vi "Kinesis-Microestruturacao-Circuits.vi"() -> ()   [LabVIEW 2014]
doc: "André Romero - 2017\nandretec@ifsc.usp.br"
uses:
  C:/UserLab/andre/GITs/andretec/Thorlabs-Vector-Move/kinesisTec/Kinesis/Thorlabs.MotionControl.Controls.dll
  Kinesis/Thorlabs.MotionControl.Controls.dll
  Basic-VIs/motorsGlobalVar.vi
  <vilib>/Instr/_visa.llb/VISA Configure Serial Port (Instr).vi
panel:
  in  "Raio":dbl=0.01
  in  "Density":dbl=100.0
  in  "Adjust Motors":bool
  out "Process time":string="0:00:50"
  out "Progress %":dbl(slide) scale=0.0..100.0
  out "XY Graph":cluster{"Graph X":dbl[], "Graph Y":dbl[]}(graph)
  in  "Swap XY":bool
  out "stop cronometro":bool=TRUE
  in  "Stop Button":bool
  in  "Graph Y":dbl[](array[numeric])=[0.0, 0.0, 6.6674440298507465, 6.6674440298507465, 6.6674440298507465, 6.6674440298507465, 6.6674440298507465, 6.6674440298507465, 6.6674440298507465, 6.6674440298507465, 6.6674440298507465, 6.6674440298507465, 6.6674440298507465, 6.6674440298507465, 6.6674440298507465, 6.6674440298507465, 6.6674440298507465, 6.6674440298507465, 6.6674440298507465, 6.6674440298507465, 6.6674440298507465, 6.6674440298507465, 6.6674440298507465, 6.6674440298507465, 6.6674440298507465, 6.6674440298507465, 6.6674440298507465, 6.6674440298507465, 6.6674440298507465, 6.6674440298507465, 6.6674440298507465, 6.6674440298507465, 6.6674440298507465, 6.6674440298507465, 6.6674440298507465, 6.6674440298507465, 6.6674440298507465, 6.6674440298507465, 6.6674440298507465, 6.6674440298507465, 6.6674440298507465, 6.6674440298507465, 6.6674440298507465, 6.673128498134329, 6.673128498134329, 6.673128498134329, 6.673128498134329, 6.673128498134329, 6.687354244402985, 6.687354244402985, 6.687354244402985, 6.687354244402985, 6.687354244402985, 6.692543143656716, 6.692543143656716, 6.692543143656716, 6.692543143656716, 6.692543143656716, 6.692543143656716, 6.692543143656716, 6.692543143656716, 6.692543143656716, 6.692543143656716, 6.692543143656716, 6.692543143656716, 6.691522854477612, 6.691522854477612, 6.691522854477612, 6.691522854477612, 6.691522854477612, 6.680183069029851, 6.680183069029851, 6.680183069029851, 6.680183069029851, 6.680183069029851, 6.658640391791045, 6.658640391791045, 6.658640391791045, 6.658640391791045, 6.658640391791045, 6.644793610074627, 6.644793610074627, 6.644793610074627, 6.644793610074627, 6.644793610074627, 6.642490671641791, 6.642490671641791, 6.642490671641791, 6.642490671641791, 6.642490671641791, 6.642490671641791, 6.642490671641791, 6.642490671641791, 6.642490671641791, 6.642490671641791, 6.642490671641791, 6.642490671641791, 6.642490671641791, 6.642490671641791, 6.642490671641791, 6.647825326492537, 6.647825326492537, 6.647825326492537, 6.647825326492537, 6.647825326492537, 6.66543260261194, 6.66543260261194, 6.66543260261194, 6.66543260261194, 6.66543260261194, 6.685226212686567, 6.685226212686567, 6.685226212686567, 6.685226212686567, 6.685226212686567, 6.692484841417911, 6.692484841417911, 6.692484841417911, 6.692484841417911, 6.692484841417911, 6.692543143656716, 6.692543143656716, 6.692543143656716, 6.692543143656716, 6.692543143656716, 6.692543143656716, 6.692543143656716, 6.691464552238806, 6.691464552238806, 6.691464552238806, 6.691464552238806, 6.691464552238806, 6.679833255597015, 6.679833255597015, 6.679833255597015, 6.679833255597015, 6.679833255597015, 6.658057369402985, 6.658057369402985, 6.658057369402985, 6.658057369402985, 6.658057369402985, 6.644647854477612, 6.644647854477612, 6.644647854477612, 6.644647854477612, 6.644647854477612, 6.642548973880597, 6.642548973880597, 6.642548973880597, 6.642548973880597, 6.642548973880597, 6.642519822761194, 6.642519822761194, 6.642519822761194, 6.642519822761194, 6.642519822761194, 6.642519822761194, 6.642519822761194, 6.642519822761194, 6.643569263059701, 6.643569263059701, 6.643569263059701, 6.643569263059701, 6.643569263059701, 6.655521222014926, 6.655521222014926, 6.655521222014926, 6.655521222014926, 6.655521222014926, 6.677180503731344, 6.677180503731344, 6.677180503731344, 6.677180503731344, 6.677180503731344, 6.690531716417911, 6.690531716417911, 6.690531716417911, 6.690531716417911, 6.690531716417911, 6.692572294776119, 6.692572294776119, 6.692572294776119, 6.692572294776119, 6.692572294776119, 6.692572294776119, 6.692572294776119, 6.692572294776119, 6.692572294776119, 6.692572294776119, 6.692572294776119, 6.692572294776119, 6.691522854477612, 6.691522854477612, 6.691522854477612, 6.691522854477612, 6.691522854477612, 6.680008162313433, 6.680008162313433, 6.680008162313433, 6.680008162313433, 6.680008162313433, 6.668668376865671, 6.668668376865671, 6.668668376865671, 6.668668376865671, 6.668668376865671, 6.667502332089552, 6.667502332089552, 6.667502332089552, 6.667502332089552, 6.667502332089552, 6.667502332089552, 6.667502332089552, 6.667502332089552, 6.667502332089552, 6.667502332089552, 6.667502332089552, 6.667502332089552, 6.667531483208955, 6.667531483208955, 6.667531483208955, 6.667531483208955, 6.667531483208955, 6.667531483208955, 6.667531483208955, 6.667531483208955, 6.667531483208955, 6.667531483208955, 6.667531483208955, 6.667531483208955, 6.667531483208955, 6.667531483208955, 6.667531483208955, 6.667531483208955, 6.667531483208955, 6.667531483208955, 6.667531483208955, 6.667531483208955, 6.667531483208955, 6.667531483208955, 6.667531483208955, 6.667531483208955, 6.667531483208955, 6.667531483208955, 6.667531483208955, 6.667531483208955, 6.667531483208955, 6.667531483208955, 6.667531483208955, 6.667531483208955, 6.667531483208955, 6.667531483208955, 6.667531483208955, 6.667531483208955, 6.667531483208955, 6.6663945895522385, 6.6663945895522385, 6.6663945895522385, 6.6663945895522385, 6.6663945895522385, 6.662051072761194, 6.662051072761194, 6.662051072761194, 6.662051072761194, 6.662051072761194, 6.644035680970149, 6.644035680970149, 6.644035680970149, 6.644035680970149, 6.644035680970149, 6.606430736940299, 6.606430736940299, 6.606430736940299, 6.606430736940299, 6.606430736940299, 6.593924906716418, 6.593924906716418, 6.593924906716418, 6.593924906716418, 6.593924906716418, 6.574539412313433, 6.574539412313433, 6.574539412313433, 6.574539412313433, 6.574539412313433, 6.567484841417911, 6.567484841417911, 6.567484841417911, 6.567484841417911, 6.567484841417911, 6.567484841417911, 6.567484841417911, 6.567484841417911, 6.567484841417911, 6.567484841417911, 6.567484841417911, 6.567513992537314, 6.567513992537314, 6.567513992537314, 6.567513992537314, 6.567513992537314, 6.567513992537314, 6.567513992537314, 6.567513992537314, 6.567513992537314, 6.567513992537314, 6.567543143656716, 6.567543143656716, 6.567543143656716, 6.567543143656716, 6.567543143656716, 6.567543143656716, 6.567543143656716, 6.567543143656716, 6.567543143656716, 6.567543143656716, 6.567543143656716, 6.567543143656716, 6.567543143656716, 6.567543143656716, 6.567543143656716, 6.567543143656716, 6.567543143656716, 6.567543143656716, 6.567543143656716, 6.567543143656716, 6.567543143656716, 6.567543143656716, 6.567543143656716, 6.567543143656716, 6.567543143656716, 6.567543143656716, 6.567543143656716, 6.567543143656716, 6.567543143656716, 6.567543143656716, 6.567543143656716, 6.567543143656716, 6.567543143656716, 6.567543143656716, 6.567543143656716, 6.567543143656716, 6.567543143656716, 6.567543143656716, 6.567543143656716, 6.567543143656716, 6.567543143656716, 6.567543143656716, 6.567543143656716, 6.567543143656716, 6.567543143656716, 6.567543143656716, 6.567543143656716, 6.567543143656716, 6.567543143656716, 6.567543143656716, 6.567543143656716, 6.567543143656716, 6.567543143656716, 6.567543143656716, 6.5667852145522385, 6.5667852145522385, 6.5667852145522385, 6.5667852145522385, 6.5667852145522385, 6.555299673507463, 6.555299673507463, 6.555299673507463, 6.555299673507463, 6.555299673507463, 6.533523787313433, 6.533523787313433, 6.533523787313433, 6.533523787313433, 6.533523787313433, 6.525186567164179, 6.525186567164179, 6.525186567164179, 6.525186567164179, 6.525186567164179, 6.517490671641791, 6.517490671641791, 6.517490671641791, 6.517490671641791, 6.517490671641791, 6.517490671641791, 6.517490671641791, 6.517490671641791, 6.517490671641791, 6.517490671641791, 6.517519822761194, 6.517519822761194, 6.517519822761194, 6.517519822761194, 6.517519822761194, 6.517519822761194, 6.517519822761194, 6.517519822761194, 6.517519822761194, 6.517519822761194, 6.517548973880597, 6.517548973880597, 6.517548973880597, 6.517548973880597, 6.517548973880597, 6.517548973880597, 6.517548973880597, 6.517548973880597, 6.517548973880597, 6.517548973880597, 6.517548973880597, 6.517548973880597, 6.517548973880597, 6.517548973880597, 6.517548973880597, 6.517548973880597, 6.517548973880597, 6.517548973880597, 6.517548973880597, 6.517548973880597, 6.517548973880597, 6.517548973880597, 6.517548973880597, 6.517548973880597, 6.517548973880597, 6.517548973880597, 6.517548973880597, 6.517548973880597, 6.517548973880597, 6.517548973880597, 6.517548973880597, 6.517548973880597, 6.517548973880597, 6.517548973880597, 6.517548973880597, 6.517548973880597, 6.517548973880597, 6.517548973880597, 6.517548973880597, 6.517548973880597, 6.517548973880597, 6.517548973880597, 6.517548973880597, 6.517548973880597, 6.517548973880597, 6.517548973880597, 6.517548973880597, 6.517548973880597, 6.517548973880597, 6.517548973880597, 6.517548973880597, 6.517548973880597, 6.517548973880597, 6.517548973880597, 6.517548973880597, 6.517548973880597, 6.517548973880597, 6.517548973880597, 6.517548973880597, 6.517548973880597, 6.516674440298507, 6.516674440298507, 6.516674440298507, 6.516674440298507, 6.516674440298507, 6.504897388059701, 6.504897388059701, 6.504897388059701, 6.504897388059701, 6.504897388059701, 6.481926305970149, 6.481926305970149, 6.481926305970149, 6.481926305970149, 6.481926305970149, 6.456943796641791, 6.456943796641791, 6.456943796641791, 6.456943796641791, 6.456943796641791, 6.4330690298507465, 6.4330690298507465, 6.4330690298507465, 6.4330690298507465, 6.4330690298507465, 6.419717817164179, 6.419717817164179, 6.419717817164179, 6.419717817164179, 6.419717817164179, 6.417473180970149, 6.417473180970149, 6.417473180970149, 6.417473180970149, 6.417473180970149, 6.417473180970149]
  in  "Graph X":dbl[](array[numeric])=[0.0, 0.0, 3.605935167910448, 3.605935167910448, 3.605935167910448, 3.605935167910448, 3.605935167910448, 3.609987173507463, 3.609987173507463, 3.609987173507463, 3.609987173507463, 3.609987173507463, 3.627157182835821, 3.627157182835821, 3.627157182835821, 3.627157182835821, 3.627157182835821, 3.6520813899253732, 3.6520813899253732, 3.6520813899253732, 3.6520813899253732, 3.6520813899253732, 3.6770930503731343, 3.6770930503731343, 3.6770930503731343, 3.6770930503731343, 3.6770930503731343, 3.697323927238806, 3.697323927238806, 3.697323927238806, 3.697323927238806, 3.697323927238806, 3.705311333955224, 3.705311333955224, 3.705311333955224, 3.705311333955224, 3.705311333955224, 3.705311333955224, 3.705311333955224, 3.705311333955224, 3.705311333955224, 3.705311333955224, 3.705311333955224, 3.7063024720149254, 3.7063024720149254, 3.7063024720149254, 3.7063024720149254, 3.7063024720149254, 3.7175839552238807, 3.7175839552238807, 3.7175839552238807, 3.7175839552238807, 3.7175839552238807, 3.7291861007462686, 3.7291861007462686, 3.7291861007462686, 3.7291861007462686, 3.7291861007462686, 3.7303521455223883, 3.7303521455223883, 3.7303521455223883, 3.7303521455223883, 3.7303521455223883, 3.7303521455223883, 3.7303521455223883, 3.7303521455223883, 3.7303521455223883, 3.7303521455223883, 3.7303521455223883, 3.7303521455223883, 3.7366779384328357, 3.7366779384328357, 3.7366779384328357, 3.7366779384328357, 3.7366779384328357, 3.7554221082089554, 3.7554221082089554, 3.7554221082089554, 3.7554221082089554, 3.7554221082089554, 3.774137126865672, 3.774137126865672, 3.774137126865672, 3.774137126865672, 3.774137126865672, 3.7803463152985075, 3.7803463152985075, 3.7803463152985075, 3.7803463152985075, 3.7803463152985075, 3.7803463152985075, 3.7803463152985075, 3.7803463152985075, 3.7803463152985075, 3.7803463152985075, 3.7803463152985075, 3.7803463152985075, 3.7803463152985075, 3.7803463152985075, 3.7803463152985075, 3.781803871268657, 3.781803871268657, 3.781803871268657, 3.781803871268657, 3.781803871268657, 3.7941930970149254, 3.7941930970149254, 3.7941930970149254, 3.7941930970149254, 3.7941930970149254, 3.816027285447761, 3.816027285447761, 3.816027285447761, 3.816027285447761, 3.816027285447761, 3.828678871268657, 3.828678871268657, 3.828678871268657, 3.828678871268657, 3.828678871268657, 3.8303404850746268, 3.8303404850746268, 3.8303404850746268, 3.8303404850746268, 3.8303404850746268, 3.8303404850746268, 3.8303404850746268, 3.8303404850746268, 3.8303404850746268, 3.8303404850746268, 3.8303404850746268, 3.8303404850746268, 3.8368703358208953, 3.8368703358208953, 3.8368703358208953, 3.8368703358208953, 3.8368703358208953, 3.8447994402985075, 3.8447994402985075, 3.8447994402985075, 3.8447994402985075, 3.8447994402985075, 3.866633628731343, 3.866633628731343, 3.866633628731343, 3.866633628731343, 3.866633628731343, 3.8803346548507465, 3.8803346548507465, 3.8803346548507465, 3.8803346548507465, 3.8803346548507465, 3.8803346548507465, 3.8803346548507465, 3.8803346548507465, 3.8803346548507465, 3.8803346548507465, 3.8803346548507465, 3.8803346548507465, 3.8803346548507465, 3.8803346548507465, 3.8803346548507465, 3.8803346548507465, 3.8803346548507465, 3.8803346548507465, 3.886631296641791, 3.886631296641791, 3.886631296641791, 3.886631296641791, 3.886631296641791, 3.9054046175373136, 3.9054046175373136, 3.9054046175373136, 3.9054046175373136, 3.9054046175373136, 3.92411963619403, 3.92411963619403, 3.92411963619403, 3.92411963619403, 3.92411963619403, 3.9303288246268657, 3.9303288246268657, 3.9303288246268657, 3.9303288246268657, 3.9303288246268657, 3.9303288246268657, 3.9303288246268657, 3.9303288246268657, 3.9303288246268657, 3.9303288246268657, 3.9303288246268657, 3.9303288246268657, 3.9303288246268657, 3.9303288246268657, 3.9303288246268657, 3.9303288246268657, 3.9303288246268657, 3.936800373134328, 3.936800373134328, 3.936800373134328, 3.936800373134328, 3.936800373134328, 3.9445545708955225, 3.9445545708955225, 3.9445545708955225, 3.9445545708955225, 3.9445545708955225, 3.95536963619403, 3.95536963619403, 3.95536963619403, 3.95536963619403, 3.95536963619403, 3.95536963619403, 3.95536963619403, 3.95536963619403, 3.95536963619403, 3.95536963619403, 3.95536963619403, 3.95536963619403, 3.956652285447761, 3.956652285447761, 3.956652285447761, 3.956652285447761, 3.956652285447761, 3.961141557835821, 3.961141557835821, 3.961141557835821, 3.961141557835821, 3.961141557835821, 3.9795067630597014, 3.9795067630597014, 3.9795067630597014, 3.9795067630597014, 3.9795067630597014, 4.004518423507463, 4.004518423507463, 4.004518423507463, 4.004518423507463, 4.004518423507463, 4.0406366604477615, 4.0406366604477615, 4.0406366604477615, 4.0406366604477615, 4.0406366604477615, 4.048624067164179, 4.048624067164179, 4.048624067164179, 4.048624067164179, 4.048624067164179, 4.0553579757462686, 4.0553579757462686, 4.0553579757462686, 4.0553579757462686, 4.0553579757462686, 4.0553579757462686, 4.0553579757462686, 4.055387126865671, 4.055387126865671, 4.055387126865671, 4.055387126865671, 4.055387126865671, 4.055387126865671, 4.055387126865671, 4.055387126865671, 4.055387126865671, 4.055387126865671, 4.0553579757462686, 4.0553579757462686, 4.0553579757462686, 4.0553579757462686, 4.0553579757462686, 4.0553579757462686, 4.0553579757462686, 4.0553579757462686, 4.0553579757462686, 4.0553579757462686, 4.0553579757462686, 4.0553579757462686, 4.0553579757462686, 4.0553579757462686, 4.0553579757462686, 4.0553579757462686, 4.0553579757462686, 4.0553579757462686, 4.0553579757462686, 4.0553579757462686, 4.0553579757462686, 4.0553579757462686, 4.0553579757462686, 4.0553579757462686, 4.0553579757462686, 4.0553579757462686, 4.0553579757462686, 4.0553579757462686, 4.0553579757462686, 4.0553579757462686, 4.0553579757462686, 4.061800373134329, 4.061800373134329, 4.061800373134329, 4.061800373134329, 4.061800373134329, 4.06972947761194, 4.06972947761194, 4.06972947761194, 4.06972947761194, 4.06972947761194, 4.091534514925373, 4.091534514925373, 4.091534514925373, 4.091534514925373, 4.091534514925373, 4.105352145522388, 4.105352145522388, 4.105352145522388, 4.105352145522388, 4.105352145522388, 4.105381296641791, 4.105381296641791, 4.105381296641791, 4.105381296641791, 4.105381296641791, 4.105381296641791, 4.105381296641791, 4.1050897854477615, 4.1050897854477615, 4.1050897854477615, 4.1050897854477615, 4.1050897854477615, 4.0951784048507465, 4.0951784048507465, 4.0951784048507465, 4.0951784048507465, 4.0951784048507465, 4.073489972014926, 4.073489972014926, 4.073489972014926, 4.073489972014926, 4.073489972014926, 4.060954990671642, 4.060954990671642, 4.060954990671642, 4.060954990671642, 4.060954990671642, 4.023874766791045, 4.023874766791045, 4.023874766791045, 4.023874766791045, 4.023874766791045, 4.008687033582089, 4.008687033582089, 4.008687033582089, 4.008687033582089, 4.008687033582089, 4.005363805970149, 4.005363805970149, 4.005363805970149, 4.005363805970149, 4.005363805970149, 4.005363805970149, 4.005363805970149, 4.005363805970149, 4.005363805970149, 4.005363805970149, 4.005363805970149, 4.005363805970149, 4.005363805970149, 4.005363805970149, 4.005363805970149, 4.005363805970149, 4.005363805970149, 4.005392957089552, 4.005392957089552, 4.005392957089552, 4.005392957089552, 4.005392957089552, 4.005392957089552, 4.005392957089552, 4.005392957089552, 4.005392957089552, 4.005392957089552, 4.005392957089552, 4.005392957089552, 4.005392957089552, 4.005392957089552, 4.005392957089552, 4.005392957089552, 4.005392957089552, 4.005392957089552, 4.005392957089552, 4.005392957089552, 4.011631296641791, 4.011631296641791, 4.011631296641791, 4.011631296641791, 4.011631296641791, 4.019472947761194, 4.019472947761194, 4.019472947761194, 4.019472947761194, 4.019472947761194, 4.042852145522388, 4.042852145522388, 4.042852145522388, 4.042852145522388, 4.042852145522388, 4.080398787313433, 4.080398787313433, 4.080398787313433, 4.080398787313433, 4.080398787313433, 4.099113805970149, 4.099113805970149, 4.099113805970149, 4.099113805970149, 4.099113805970149, 4.103777985074627, 4.103777985074627, 4.103777985074627, 4.103777985074627, 4.103777985074627, 4.105410447761194, 4.105410447761194, 4.105410447761194, 4.105410447761194, 4.105410447761194, 4.105410447761194, 4.105410447761194, 4.105410447761194, 4.105381296641791, 4.105381296641791, 4.105381296641791, 4.105381296641791, 4.105381296641791, 4.098297574626866, 4.098297574626866, 4.098297574626866, 4.098297574626866, 4.098297574626866, 4.089989505597015, 4.089989505597015, 4.089989505597015, 4.089989505597015, 4.089989505597015, 4.06083838619403, 4.06083838619403, 4.06083838619403, 4.06083838619403, 4.06083838619403, 4.0553579757462686, 4.0553579757462686, 4.0553579757462686, 4.0553579757462686, 4.0553579757462686, 4.0553579757462686, 4.0553579757462686, 4.0553579757462686, 4.0553579757462686, 4.0553579757462686, 4.0553579757462686, 4.0553579757462686, 4.055387126865671, 4.055387126865671, 4.055387126865671, 4.055387126865671, 4.055387126865671, 4.055416277985074, 4.055416277985074, 4.055416277985074, 4.055416277985074, 4.055416277985074, 4.055416277985074, 4.055416277985074, 4.055416277985074, 4.055416277985074, 4.055416277985074, 4.055416277985074, 4.055416277985074, 4.055416277985074, 4.055416277985074, 4.055416277985074, 4.055416277985074, 4.055416277985074, 4.055416277985074, 4.055416277985074, 4.055416277985074, 4.055416277985074, 4.055416277985074, 4.055416277985074, 4.055416277985074, 4.055416277985074, 4.055416277985074, 4.055416277985074, 4.055416277985074, 4.055416277985074, 4.055416277985074, 4.055416277985074]
  out "GetPOS Y":dbl=6.417473180970149 format="%_6f"
  out "GetPOS X":dbl=4.055416277985074 format="%#_6f"
  out ".NET Refnum out 2":refnum<k24>
  out ".NET Refnum out 1":refnum<k24>
  out "Motor 2":bool
  out "Motor 1":bool
  in  "Acceleration (mm/s)":dbl=0.05
  in  "Iniciar":bool
  in  "Velocity (mm/s)":sgl=0.05
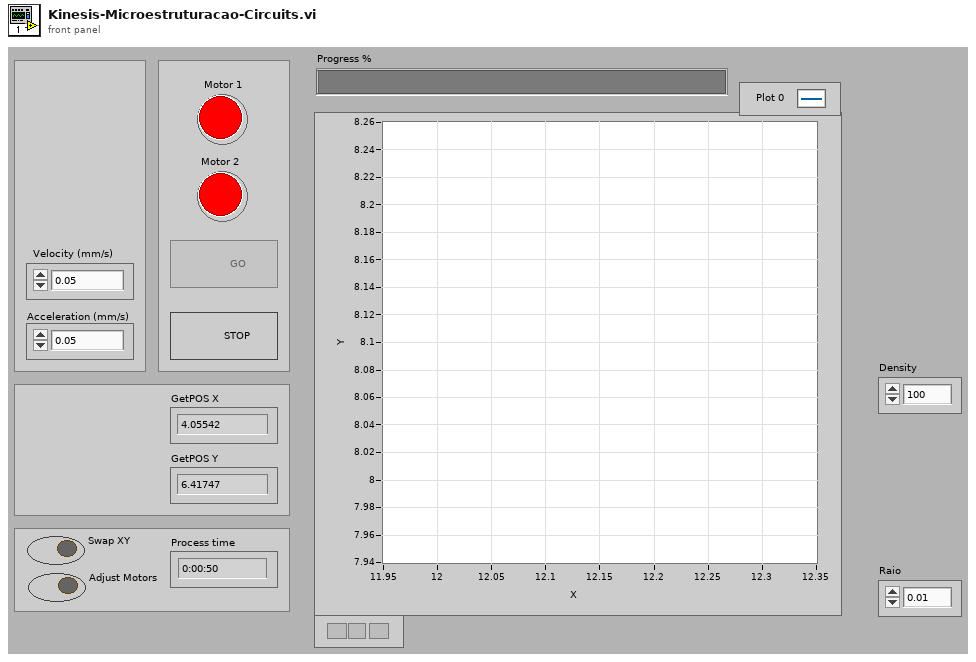
[diagram p1: front panel]
types:
  T1 = enum8{"Enabled", "Disabled", "Disabled and Grayed Out"}
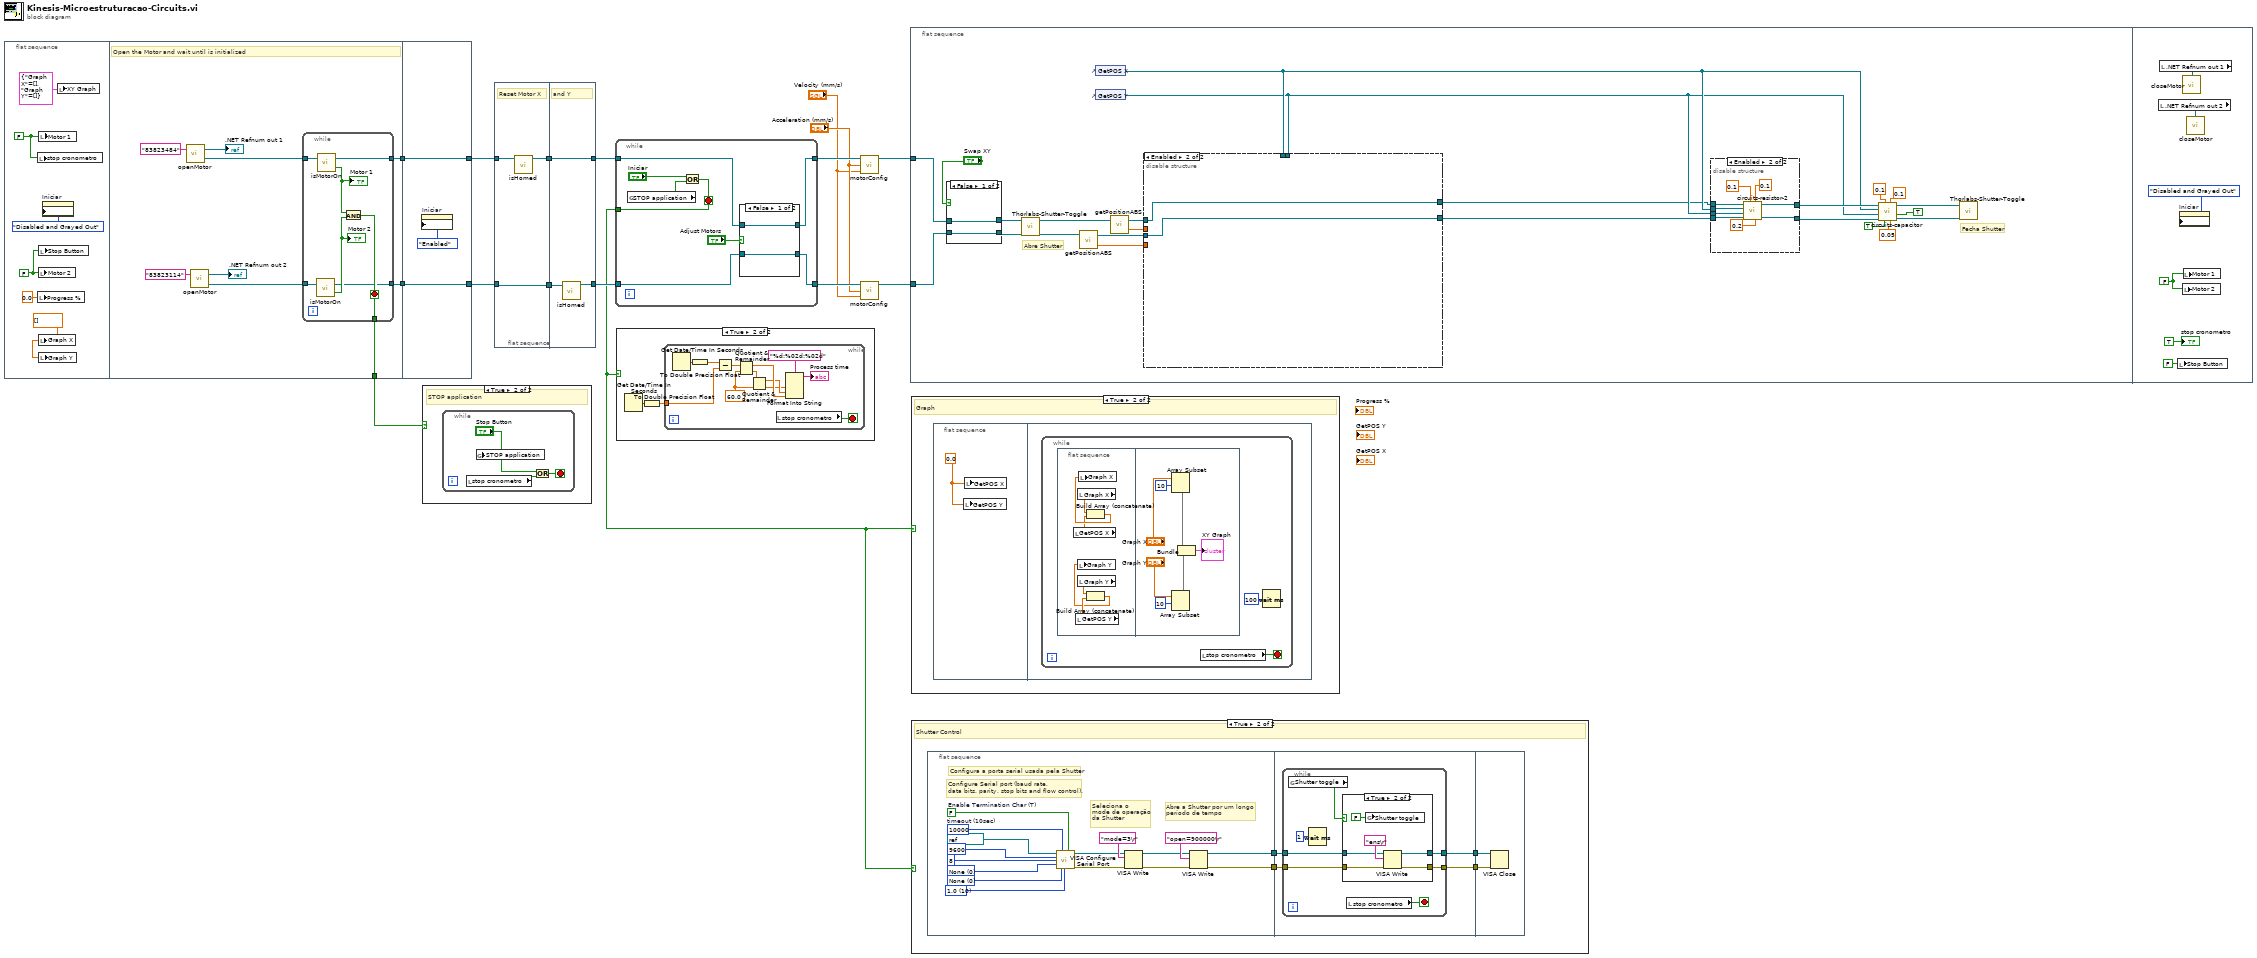
[diagram p0: block diagram]
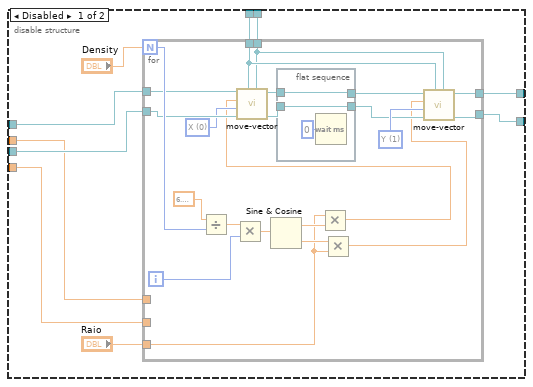
[diagram p6: hidden frame]
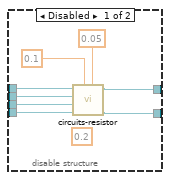
[diagram p7: hidden frame]
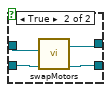
[diagram p8: hidden frame]
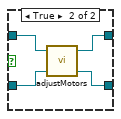
[diagram p10: hidden frame]
diagram:
  n1 = flat-sequence {
    tunnel: [w31] -> w4
    tunnel: [w30] -> w3
    tunnel: [w29] -> w2
    tunnel: [w40] -> w7
    tunnel: [w41] -> w8
    tunnel: w4 -> [w41]
    tunnel: w3 -> [w40]
    frame #0 {
      w18 = dbl[] [] ("Graph Y")
      w21 = FALSE ("Motor3\nLigado")
      w22 = FALSE
      n2 = local write "stop cronometro"(w22) -> ()
      n3 = local write "Progress %"(0.0 ("Progress %")) -> ()
      n4 = local write "Motor 2"(w21) -> ()
      n5 = local write "Graph X"(w18) -> ()
      n6 = local write "Motor 1"(w22) -> ()
      n7 = local write "Stop Button"(w21) -> ()
      n8 = local write "Graph Y"(w18) -> ()
      n9 = property on="Iniciar" class="Bool (strict)"("DisabledEnum"=T1."Disabled and Grayed Out" ("Disabled")) -> ()  [unwired: 2 in, 2 out]
      n10 = local write "XY Graph"(cluster{"Graph X":dbl[], "Graph Y":dbl[]} {"Graph X"=[], "Graph Y"=[]} ("XY Graph")) -> ()
    }
    frame #1 {
      # "Open the Motor and wait until is initialized"
      n11 = call "openMotor.vi"("S/N Motor"="83823484") -> ("Device"=w27:refnum<k24>, ".NET Refnum out"=→".NET Refnum out 1":refnum<k24>)  [unwired: 1 in]
      n12 = call "openMotor.vi"("S/N Motor"="83823114") -> ("Device"=w28:refnum<k24>, ".NET Refnum out"=→".NET Refnum out 2":refnum<k24>)  [unwired: 1 in]
      n13 = while {
        tunnel: w27 -> [w36]
        tunnel: w28 -> [w35]
        tunnel: [w33] -> w31
        tunnel: [w32] -> w30
        tunnel: [w34] -> w29
        stop <- w34 stop-if-true
        n14 = call "isMotorOn.vi"("Device"=w35) -> ("isConnected"=w37:bool, "Device out"=w32:refnum<k24>)  [unwired: 1 in]
        "Motor 2" <- w37
        n15 = call "isMotorOn.vi"("Device"=w36) -> ("isConnected"=w38:bool, "Device out"=w33:refnum<k24>)  [unwired: 1 in]
        "Motor 1" <- w38
        n16 = And(x=w38, y=w37) -> (x .and. y?=w34:bool)
      }
    }
    frame #2 {
      n17 = property on="Iniciar" class="Bool (strict)"("DisabledEnum"=T1."Enabled" ("Disabled")) -> ()  [unwired: 2 in, 2 out]
    }
  }
  n18 = case shown="True" w2 {
    frame False {
    }
    frame True {
      # "STOP application"
      n19 = while {
        stop <- w43 stop-if-true
        n20 = local read "stop cronometro"() -> (w42:bool)
        n21 = global write "motorsGlobalVar.vi" "STOP application"("Stop Button") -> ()
        n22 = Or(x="Stop Button", y=w42) -> (x .or. y?=w43:bool)
      }
    }
  }
  n23 = flat-sequence {
    tunnel: w8 -> [w47]
    tunnel: w7 -> [w45]
    tunnel: [w46] -> w6
    tunnel: [w45] -> w5
    tunnel: [w50] -> w10
    tunnel: [w49] -> w9
    tunnel: w6 -> [w50]
    tunnel: w5 -> [w48]
    frame #0 {
      # "Reset Motor X"
      n24 = call "isHomed.vi"("Device in"=w47) -> ("Device out"=w46:refnum<k24>)  [unwired: 4 in]
    }
    frame #1 {
      # "and Y"
      n25 = call "isHomed.vi"("Device in"=w48) -> ("Device out"=w49:refnum<k24>)  [unwired: 4 in]
    }
  }
  n26 = while {
    tunnel: [w58] -> w1
    tunnel: w10 -> [w53]
    tunnel: w9 -> [w54]
    tunnel: [w52] -> w16
    tunnel: [w51] -> w15
    stop <- w58 stop-if-true
    n27 = global read "motorsGlobalVar.vi" "STOP application"() -> (w56:bool)
    n28 = Or(x="Iniciar", y=w56) -> (x .or. y?=w58:bool)
    n29 = case shown="False" "Adjust Motors" {
      tunnel: w54 -> [w59 w64]
      tunnel: w53 -> [w60 w63]
      tunnel: [w60 w62] -> w52
      tunnel: [w59 w61] -> w51
      frame False {
      }
      frame True {
        n30 = call "adjustMotors.vi"("Device 2"=w64, "Device 1"=w63) -> ("Device out 2"=w61:refnum<k24>, "Device out 1"=w62:refnum<k24>)  [unwired: 2 in]
      }
    }
  }
  n31 = case shown="True" w1 {
    frame False {
    }
    frame True {
      n32 = Get Date/Time In Seconds() -> (seconds since 1Jan1904=w66:timestamp)
      n33 = To Double Precision Float(number=w66) -> (double precision float=w65:dbl)
      n34 = while {
        tunnel: w65 -> [w70]
        stop <- w78 stop-if-true
        w75 = 60.0 ("y")
        n35 = Get Date/Time In Seconds() -> (seconds since 1Jan1904=w77:timestamp)
        n36 = To Double Precision Float(number=w77) -> (double precision float=w71:dbl)
        n37 = Subtract(x=w71, y=w70) -> (x-y=w69:dbl)
        n38 = Quotient & Remainder(x=w69, y=w75) -> (x-y*floor(x/y)=w74:dbl, floor(x/y)=w76:dbl)
        n39 = Quotient & Remainder(x=w76, y=w75) -> (x-y*floor(x/y)=w73:dbl, floor(x/y)=w72:dbl)
        n40 = local read "stop cronometro"() -> (w78:bool)
        n41 = Format Into String(format string="%d:%02d:%02d", w72, w73, w74) -> (resulting string=→"Process time":string)  [unwired: 2 in, 1 out]
      }
    }
  }
  n42 = call "motorConfig.vi"("Velocity"="Velocity (mm/s)", "Acceleration"="Acceleration (mm/s)", "Device in"=w16) -> ("Device out"=w12:refnum<k24>)  [unwired: 2 in]
  n43 = call "motorConfig.vi"("Velocity"="Velocity (mm/s)", "Acceleration"="Acceleration (mm/s)", "Device in"=w15) -> ("Device out"=w11:refnum<k24>)  [unwired: 2 in]
  n44 = flat-sequence {
    tunnel: w12 -> [w102]
    tunnel: w11 -> [w101]
    frame #0 {
      # "Fecha Shutter"
      # "Abre Shutter"
      n45 = case shown="False" "Swap XY" {
        tunnel: w102 -> [w158 w162]
        tunnel: w101 -> [w157 w161]
        tunnel: [w158 w160] -> w97
        tunnel: [w157 w159] -> w96
        frame False {
        }
        frame True {
          n46 = call "swapMotors.vi"("Device 2"=w161, "Device 1"=w162) -> ("Device out 1"=w159:refnum<k24>, "Device out 2"=w160:refnum<k24>)  [unwired: 2 in, 2 out]
        }
      }
      n47 = call "Thorlabs-Shutter-Toggle.vi"("Device in Y"=w96, "Device in X"=w97) -> ("Device out Y"=w86:refnum<k24>, "Device out X"=w88:refnum<k24>)  [unwired: 8 in]
      n48 = call "getPositionABS.vi"("Device"=w86) -> ("GetPOS"=w83:dbl, "Device out"=w85:refnum<k24>)  [unwired: 1 in]
      n49 = control-ref of="GetPOS X"() -> (w82:refnum<vi>)
      n50 = control-ref of="GetPOS Y"() -> (w81:refnum<vi>)
      n51 = call "getPositionABS.vi"("Device"=w88) -> ("GetPOS"=w84:dbl, "Device out"=w87:refnum<k24>)  [unwired: 1 in]
      n52 = disable-structure shown="Enabled" {
        disable-tunnel: w87 -> [w110 w139]
        disable-tunnel: w85 -> [w109 w138]
        disable-tunnel: w84 -> [w108 _]
        disable-tunnel: w83 -> [w107 _]
        disable-tunnel: w82 -> [w106 _]
        disable-tunnel: w81 -> [w105 _]
        disable-tunnel: [w104 w139] -> w80
        disable-tunnel: [w103 w138] -> w79
        frame Disabled {
          n53 = for {
            N: "Density" -> [w129]
            tunnel: w108 -> [_]
            tunnel: w107 -> [_]
            tunnel: "Raio" -> [w127]
            tunnel: w110 -> [w126]
            tunnel: w109 -> [w125]
            tunnel: w106 -> [w120]
            tunnel: w105 -> [w119]
            tunnel: [w122] -> w104
            tunnel: [w121] -> w103
            i -> [w128]
            w123 = u16 1 items=["X", "Y"] ("X-Y")
            w124 = u16 0 items=["X", "Y"] ("X-Y")
            n54 = Divide(x=6.283185307179586, y=w129) -> (x/y=w134:dbl)
            n55 = Multiply(x=w134, y=w128) -> (x*y=w133:dbl)
            n56 = Sine & Cosine(0:w133) -> (1:w132:dbl, 2:w131:dbl)
            n57 = flat-sequence {
              tunnel: w118 -> [w137]
              tunnel: [w137] -> w115
              tunnel: w117 -> [w136]
              tunnel: [w136] -> w116
              frame #0 {
                n58 = Wait (ms)(milliseconds to wait=u32 0) -> ()  [unwired: 1 out]
              }
            }
            n59 = Multiply(x=w127, y=w132) -> (x*y=w114:dbl)
            n60 = call "move-vector.vi"("GetPOS Y"=w119, "GetPOS X"=w120, "Device in Y"=w125, "X-Y"=w124, "Distance"=w114, "Device in X"=w126) -> ("Device out Y"=w117:refnum<k24>, "Device out X"=w118:refnum<k24>)  [unwired: 4 in]
            n61 = Multiply(x=w131, y=w127) -> (x*y=w113:dbl)
            n62 = call "move-vector.vi"("GetPOS Y"=w119, "GetPOS X"=w120, "Device in Y"=w116, "X-Y"=w123, "Distance"=w113, "Device in X"=w115) -> ("Device out Y"=w121:refnum<k24>, "Device out X"=w122:refnum<k24>)  [unwired: 4 in]
          }
        }
        frame Enabled {
        }
      }
      n63 = disable-structure shown="Enabled" {
        disable-tunnel: [w145 w152] -> w99
        disable-tunnel: [w144 w151] -> w98
        disable-tunnel: w82 -> [w143 w154]
        disable-tunnel: w81 -> [w142 w153]
        disable-tunnel: w80 -> [w141 w156]
        disable-tunnel: w79 -> [w140 w155]
        frame Disabled {
          (unwired) 0.2 ("L3")
          n64 = call "circuits-resistor.vi"("L2"=0.05, "L1"=0.1, "Device in Y"=w140, "GetPOS Y"=w142, "GetPOS X"=w143, "Device in X"=w141) -> ("Device out Y"=w144:refnum<k24>, "Device out X"=w145:refnum<k24>)  [unwired: 4 in]
        }
        frame Enabled {
          n65 = call "circuits-resistor-2.vi"("L3"=0.2, "L2"=0.1, "L1"=0.1, "Device in Y"=w155, "GetPOS Y"=w153, "GetPOS X"=w154, "Device in X"=w156) -> ("Device out Y"=w151:refnum<k24>, "Device out X"=w152:refnum<k24>)  [unwired: 3 in]
        }
      }
      n66 = call "circuits-capacitor.vi"("Invert Y"=TRUE, "L2"=0.05, "L3"=0.1, "Swap-XY"=TRUE, "L1"=0.1, "Device in Y"=w98, "GetPOS Y"=w81, "GetPOS X"=w82, "Device in X"=w99) -> ("Device out Y"=w94:refnum<k24>, "Device out X"=w95:refnum<k24>)  [unwired: 1 in]
      n67 = call "Thorlabs-Shutter-Toggle.vi"("Device in Y"=w94, "Device in X"=w95) -> ()  [unwired: 8 in, 2 out]
    }
    frame #1 {
      w166 = FALSE
      n68 = local read ".NET Refnum out 2"() -> (w167:refnum<k24>)
      n69 = local read ".NET Refnum out 1"() -> (w168:refnum<k24>)
      n70 = local write "Stop Button"(FALSE ("Stop Button")) -> ()
      n71 = property on="Iniciar" class="Bool (strict)"("DisabledEnum"=T1."Disabled and Grayed Out" ("Disabled")) -> ()  [unwired: 2 in, 2 out]
      n72 = call "closeMotor.vi"(".NET Refnum in"=w168) -> ()  [unwired: 2 in]
      n73 = local write "Motor 2"(w166) -> ()
      n74 = local write "Motor 1"(w166) -> ()
      n75 = call "closeMotor.vi"(".NET Refnum in"=w167) -> ()  [unwired: 2 in]
      "stop cronometro" <- TRUE ("stop cronometro")
    }
  }
  n76 = case shown="True" w1 {
    frame False {
    }
    frame True {
      # "Graph"
      n77 = flat-sequence {
        frame #0 {
          w169 = 0.0
          n78 = local write "GetPOS Y"(w169) -> ()
          n79 = local write "GetPOS X"(w169) -> ()
        }
        frame #1 {
          n80 = while {
            stop <- w170 stop-if-true
            n81 = flat-sequence {
              frame #0 {
                n82 = local read "GetPOS X"() -> (w175:dbl)
                n83 = local read "GetPOS Y"() -> (w174:dbl)
                n84 = local read "Graph X"() -> (w177:dbl[])
                n85 = local read "Graph Y"() -> (w172:dbl[])
                n86 = Build Array (concatenate)(w177, w175) -> (w176:dbl[])
                n87 = local write "Graph X"(w176) -> ()
                n88 = Build Array (concatenate)(w172, w174) -> (w173:dbl[])
                n89 = local write "Graph Y"(w173) -> ()
              }
              frame #1 {
                n90 = Array Subset(array="Graph Y", index=10) -> (w178:dbl[])  [unwired: 1 in]
                n91 = Array Subset(array="Graph X", index=10) -> (w181:dbl[])  [unwired: 1 in]
                n92 = Bundle(w181, w178) -> (→"XY Graph":cluster{dbl[], dbl[]})  [unwired: 1 in]
              }
            }
            n93 = local read "stop cronometro"() -> (w170:bool)
            n94 = Wait (ms)(milliseconds to wait=u32 100) -> ()  [unwired: 1 out]
          }
        }
      }
    }
  }
  n95 = case shown="True" w1 {
    frame False {
    }
    frame True {
      # "Shutter Control"
      n96 = flat-sequence {
        tunnel: [w190] -> w188
        tunnel: [w189] -> w187
        tunnel: w188 -> [w208]
        tunnel: w187 -> [w205]
        tunnel: [w207] -> w186
        tunnel: [w206] -> w185
        tunnel: w186 -> [w225]
        tunnel: w185 -> [w224]
        frame #0 {
          w200 = u16 0 items=["None", "Odd", "Even", "Mark", "Space"] ("parity")
          w197 = u16 10 items=["1.0"=10, "1.5"=15, "2.0"=20] ("stop bits")
          w196 = u16 0 items=["None"=0, "XON/XOFF"=1, "RTS/CTS"=2, "DTR/DSR"=4] ("flow control")
          w198 = FALSE  # Enable Termination Char (T)
          w199 = u32 10000  # timeout (10sec)
          # "Configura a porta serial usada pela Shutter"
          # "Configure Serial port (baud rate,\ndata bits, parity, stop bits and flow control)."
          # "Seleciona o \nmode de operação\nda Shutter"
          # "Abre a Shutter por um longo\nperíodo de tempo"
          n97 = call-poly "VISA Configure Serial Port"("VISA resource name"=refnum<visa-resource-name> "COM3", "timeout (10sec)"=w199, "Enable Termination\nChar (T)"=w198, "baud rate (9600)"=u32 9600 ("baud rate"), "data bits (8)"=u16 8 ("data bits"), "parity (0:none)"=w200, "stop bits (10: 1 bit)"=w197, "flow control (0:none)"=w196) -> ("VISA resource name out"=w194:refnum<visa-resource-name>, "error out"=w193:errorcluster)  [unwired: 6 in]
          n98 = VISA Write(VISA resource name=w194, write buffer="mode=3\r", error in (no error)=w193) -> (VISA resource name out=w192:refnum<visa-resource-name>, error out=w191:errorcluster)  [unwired: 1 out]
          n99 = VISA Write(VISA resource name=w192, write buffer="open=900000\r", error in (no error)=w191) -> (VISA resource name out=w190:refnum<visa-resource-name>, error out=w189:errorcluster)  [unwired: 1 out]
        }
        frame #1 {
          n100 = while {
            tunnel: w208 -> [w215]
            tunnel: [w214] -> w207
            tunnel: [w213] -> w206
            tunnel: w205 -> [w212]
            stop <- w209 stop-if-true
            n101 = global read "motorsGlobalVar.vi" "Shutter toggle"() -> (w211:bool)
            n102 = Wait (ms)(milliseconds to wait=u32 1) -> ()  [unwired: 1 out]
            n103 = case shown="True" w211 {
              tunnel: w215 -> [w217 w222]
              tunnel: [w217 w221] -> w214
              tunnel: [w216 w220] -> w213
              tunnel: w212 -> [w216 w219]
              frame False {
              }
              frame True {
                n104 = global write "motorsGlobalVar.vi" "Shutter toggle"(FALSE ("Shutter toggle")) -> ()
                n105 = VISA Write(VISA resource name=w222, write buffer="ens\r", error in (no error)=w219) -> (VISA resource name out=w221:refnum<visa-resource-name>, error out=w220:errorcluster)  [unwired: 1 out]
              }
            }
            n106 = local read "stop cronometro"() -> (w209:bool)
          }
        }
        frame #2 {
          n107 = VISA Close(VISA resource name=w225, error in (no error)=w224) -> ()  [unwired: 1 out]
        }
      }
    }
  }
